vi "readRecetaDataInRecetaTable.vi"(8 "error in":errorcluster, 11 "dataToQueryOfRead":T1) -> (0 "error out":errorcluster, 3 "ClusterFormat":T2)   [LabVIEW 2014]
uses:
  <vilib>/addons/database/NI_Database_API.lvlib
  <vilib>/addons/database/Connection.llb/DB Tools Open Connec (String).vi
  <vilib>/addons/database/Auxilliary.llb/DB Tools Format Datetime String (Time Stamp).vi
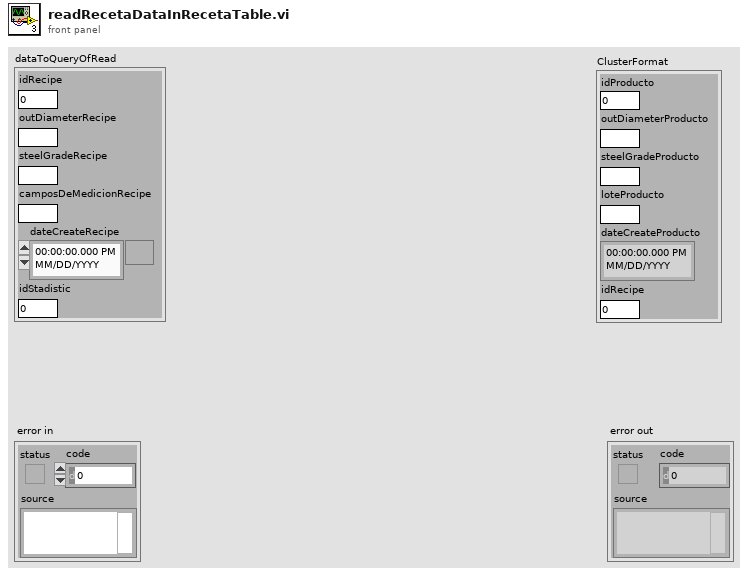
[diagram p1: front panel]
types:
  T1 = cluster{"idRecipe":dbl, "outDiameterRecipe":string, "steelGradeRecipe":string, "camposDeMedicionRecipe":string, "dateCreateRecipe":timestamp, "idStadistic":dbl}
  T2 = cluster{"idProducto":dbl, "outDiameterProducto":string, "steelGradeProducto":string, "loteProducto":string, "dateCreateProducto":timestamp, "idRecipe":dbl}
  T3 = typedef "NI_Database_API.lvlib/Conn ObjectReference.ctl" = refnum<k1>
  T4 = typedef "NI_Database_API.lvlib/DB Tools DataTypes.ctl" = enum16{"String", "Long (I32)", "Single (SGL)", "Double (DBL)", "Date/Time", "Binary"}
  T5 = cluster{"name":string, "database data type":T4, "defined size":i32}[]
  T6 = cluster{string, "outDiameterRecipe":string, "steelGradeRecipe":string, "camposDeMedicionRecipe":string, "date/time string":string, string}
  T7 = cluster{"idRod":dbl, "camposDeMedicion":string, "dateCreate":timestamp, "idProduct":dbl, "idImage":dbl}
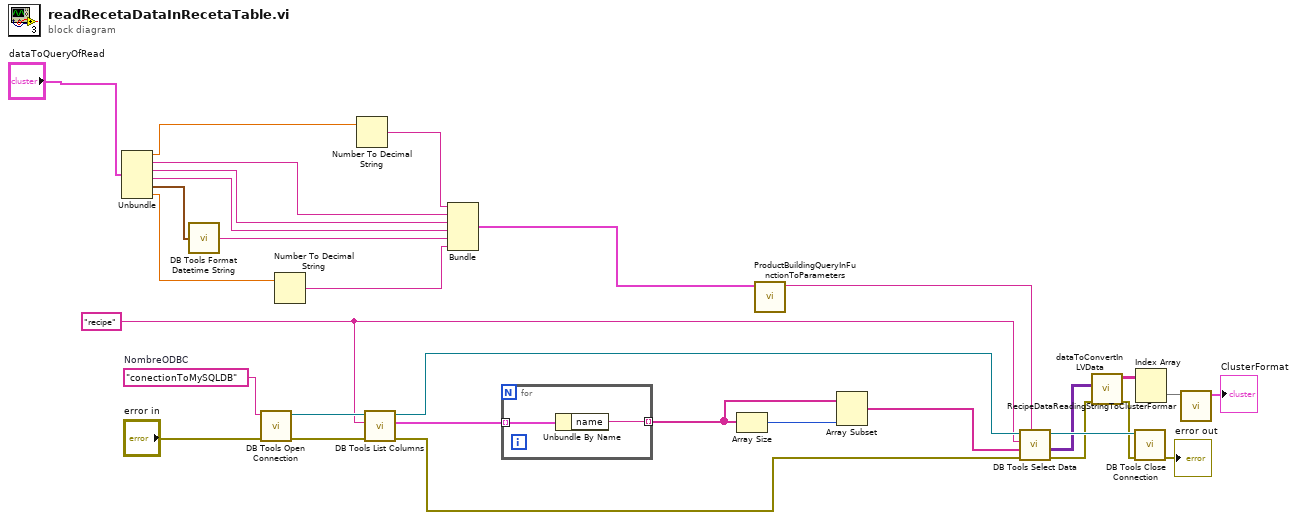
[diagram p0: block diagram]
diagram:
  w18 = "recipe" ("tableName")
  w31 = "conectionToMySQLDB"  # NombreODBC
  n1 = Unbundle("dataToQueryOfRead") -> ("idRecipe"=w25:dbl, "outDiameterRecipe"=w24:string, "steelGradeRecipe"=w7:string, "camposDeMedicionRecipe"=w6:string, "dateCreateRecipe"=w8:timestamp, "idStadistic"=w4:dbl)
  n2 = call-poly <vilib>:"DB Tools Format Datetime String.vi"("time stamp"=w8) -> ("date/time string"=w5:string)
  n3 = call-poly <vilib>:"DB Tools Open Connection.vi"("error in (no error)"="error in", "connection information"=w31) -> ("error out"=w29:errorcluster, "connection reference"=w30:T3)  [unwired: 6 in]
  n4 = Number To Decimal String(number=w4) -> (decimal integer string=w3:string)  [unwired: 1 in]
  n5 = Number To Decimal String(number=w25) -> (decimal integer string=w26:string)  [unwired: 1 in]
  n6 = call <vilib>:"DB Tools List Columns.vi"("error in (no error)"=w29, "table"=w18, "connection reference"=w30) -> ("error out"=w19:errorcluster, "column information"=w27:T5, "connection reference out"=w20:T3)  [unwired: 1 in, 1 out]
  n7 = Bundle(w26, "outDiameterRecipe"=w24, "steelGradeRecipe"=w7, "camposDeMedicionRecipe"=w6, "date/time string"=w5, w3) -> (w17:T6)  [unwired: 1 in]
  n8 = for {
    tunnel: w27 -> [w33] mode=indexing
    tunnel: [w32] -> w22 mode=indexing
    n9 = Unbundle By Name(w33) -> ("name"=w32:string)
  }
  n10 = Array Size(array=w22) -> (size(s)=w23:i32)
  n11 = call "ProductBuildingQueryInFunctionToParameters.vi"("ParameterToRead"=w17) -> ("QueryToRead"=w16:string)  [unwired: 10 in]
  n12 = Array Subset(array=w22, length=w23) -> (w21:string[])  [unwired: 1 in]
  n13 = call <vilib>:"DB Tools Select Data.vi"("condition"=w16, "error in (no error)"=w19, "columns"=w21, "table"=w18, "connection reference"=w20) -> ("error out"=w12:errorcluster, "data"=w13:variant[][], "connection reference out"=w15:T3)  [unwired: 1 in]
  n14 = call "dataToConvertInLVData.vi"("error in"=w12, "dataReadingIn"=w13) -> ("error out"=w11:errorcluster, "dataReadingOut"=w10:string[][])  [unwired: 8 in]
  n15 = call <vilib>:"DB Tools Close Connection.vi"("error in (no error)"=w11, "connection reference"=w15) -> ("error out"=→"error out":errorcluster)  [unwired: 5 in]
  n16 = Index Array(array=w10) -> (element=w9:string[])  [unwired: 2 in]
  n17 = call "RecipeDataReadingStringToClusterFormar.vi"("StringFormat"=w9) -> ("ClusterFormat"=→"ClusterFormat":T7)  [unwired: 10 in]
